vi "VCOControl-HWTimedLoop.vi"() -> ()   [LabVIEW 2014]
uses:
  <vilib>/DAQmx/create/channels.llb/DAQmx Create Channel (AI-Voltage-Basic).vi
  <vilib>/DAQmx/configure/timing.llb/DAQmx Timing (Sample Clock).vi
  <vilib>/DAQmx/read.llb/DAQmx Read (Analog Wfm 1Chan NSamp).vi
  <vilib>/DAQmx/create/channels.llb/DAQmx Create Channel (AO-Voltage-Basic).vi
  <vilib>/DAQmx/write.llb/DAQmx Write (Analog DBL 1Chan 1Samp).vi
  <vilib>/measure/NI_MAPro.lvlib
  <vilib>/measure/matone.llb/Extract Single Tone Information 1 Chan.vi
  <vilib>/addons/control/pid/NI_PID_pid.lvlib
  <vilib>/addons/control/pid/pid.llb/PID (DBL).vi
  <vilib>/platform/TimedLoop/XDataNode/XDataNode.xnode
  <vilib>/Platform/TimedLoop/XDataNode/nitl_modes.ctl
  <vilib>/Platform/TimedLoop/XDataNode/XDNodeRunTimeDep.lvlib
  <vilib>/Platform/TimedLoop/XDataNode/wakeup.ctl
  <vilib>/Platform/TimedLoop/XDataNode/timing_clust.ctl
  <vilib>/UPVI/lvhdf5/file.llb/LVH5F Operation.ctl
  <vilib>/UPVI/lvhdf5/library.llb/HDF5 Ref.ctl
  <vilib>/UPVI/lvhdf5/dataset.llb/LVH5D Operation.ctl
  <vilib>/UPVI/lvhdf5/dataset.llb/Simple OpenCreateReplace Dataset.xnode
  <vilib>/UPVI/lvhdf5/dataset.llb/Simple OpenCreateReplace Dataset (Variant).vi
  <vilib>/UPVI/lvhdf5/dataset.llb/Append Element(s) to Dataset.xnode
  <vilib>/UPVI/lvhdf5/dataset.llb/Append Element(s) to Dataset (Variant).vi
panel:
  in  "Dataset Path":string
  in  "path":path
  in  "PID gains":T1={"proportional gain (Kc)"=1.0, "integral time (Ti, min)"=0.01, "derivative time (Td, min)"=0.0} {"derivative time (Td, min)" format="%.3f"; "integral time (Ti, min)" format="%.3f"; "proportional gain (Kc)" format="%.3f"}
  in  "Setpoint Frequency":dbl format="%.2f"
  in  "stop":bool
  in  "AO Channel":tag
  in  "AI Channel":tag
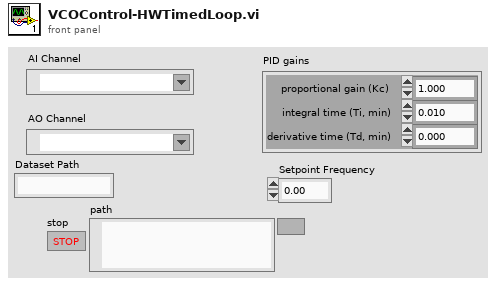
[diagram p1: front panel]
types:
  T1 = cluster{"proportional gain (Kc)":dbl, "integral time (Ti, min)":dbl, "derivative time (Td, min)":dbl}
  T2 = typedef "LVH5F Operation.ctl" = enum16{"open", "open or create", "create or replace", "create or replace (with confirmation)", "create", "open (read only)"}
  T3 = typedef "HDF5 Ref.ctl" = refnum<k1>
  T4 = typedef "XDNodeRunTimeDep.lvlib/timing_clust.ctl" = cluster{"Expected End [f-1]":u64, "Actual End [f-1]":u64, "Finished Late? [f-1]":bool, "Expected End [i-1]":u64, "Actual End [i-1]":u64, "Finished Late? [i-1]":bool, "Expected Start [i]":u64, "Actual Start [i]":u64, "Expected Start [f]":u64, "Actual Start [f]":u64, "Source Name":string, "Structure Name":string, "Period":i64, "Deadline":i64, "Offset":i64, "Start":i64, "Priority":i32, "Timeout":i32, "Mode":T5, "Wakeup Reason":T6, "Error":errorcluster, "Source Type":string, "Secondary Source Type":string, "Global End Time":u64, "Global Start Time":u64, "Frame Duration":u64, "Iteration Duration":u64, "Assigned CPU":i32, "I/O Scan Engine Mode":u32}
  T5 = typedef "XDNodeRunTimeDep.lvlib/nitl_modes.ctl" = enum32{"No Change", "Process missed periods, maintain original phase", "Discard missed periods, maintain original phase", "Process missed periods, ignore original phase", "Discard missed periods, ignore original phase"}
  T6 = typedef "XDNodeRunTimeDep.lvlib/wakeup.ctl" = enum32{"Normal", "Aborted", "Asynchronous wakeup", "Timing source error", "Timed loop error", "Timeout"}
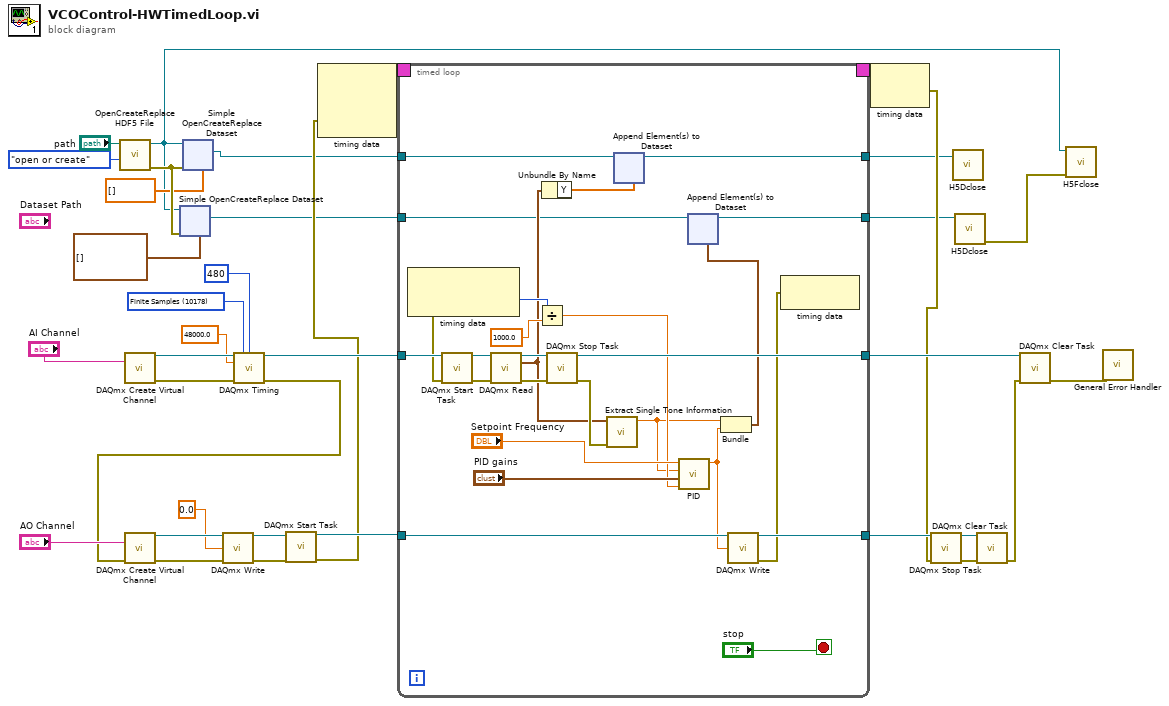
[diagram p0: block diagram]
diagram:
  w33 = 10178 items=["Finite Samples"=10178, "Continuous Samples"=10123, "Hardware Timed Single Point"=12522] ("sample mode")
  n1 = call <vilib>:"OpenCreateReplace HDF5 File.vi"("function (open or create)"=LVH5F_Operation."open or create", "path"="path") -> ("error out"=w9:errorcluster, "HDF5 Ref out"=w2:T3)  [unwired: 6 in]
  n2 = call-poly <vilib>:"DAQmx Create Virtual Channel.vi"("physical channels"="AI Channel") -> ("task out"=w35:refnum<k21>, "error out"=w34:errorcluster)  [unwired: 13 in]
  n3 = xnode "Simple OpenCreateReplace Dataset"("HDF5 Ref"=w2, "error in (no error)"=w9, "Datatype and Dataspace"=cluster{"f":dbl, "V":dbl}[] []) -> ("HDF5 Dataset Ref out"=w5:T3)  [unwired: 5 in, 2 out]
  n4 = xnode "Simple OpenCreateReplace Dataset"("HDF5 Ref"=w2, "error in (no error)"=w9, "Datatype and Dataspace"=dbl[] []) -> ("HDF5 Dataset Ref out"=w6:T3)  [unwired: 5 in, 2 out]
  n5 = call-poly <vilib>:"DAQmx Timing.vi"("task/channels in"=w35, "sample mode"=w33, "samples per channel"=480, "rate"=48000.0, "error in"=w34) -> ("task out"=w30:refnum<k21>, "error out"=w17:errorcluster)  [unwired: 9 in]
  n6 = call-poly <vilib>:"DAQmx Create Virtual Channel.vi"("physical channels"="AO Channel", "error in"=w17) -> ("task out"=w22:refnum<k21>, "error out"=w20:errorcluster)  [unwired: 12 in]
  n7 = call-poly <vilib>:"DAQmx Write.vi"("task/channels in"=w22, "data"=0.0, "error in"=w20) -> ("task out"=w21:refnum<k21>, "error out"=w19:errorcluster)  [unwired: 10 in, 1 out]
  n8 = call <vilib>:"DAQmx Start Task.vi"("task/channels in"=w21, "error in"=w19) -> ("task out"=w26:refnum<k21>, "error out"=w13:errorcluster)  [unwired: 12 in]
  n9 = node-c288(w13) -> (w15:T4)  [unwired: 2 in]
  n10 = timed-loop {
    tunnel: w30 -> [w62]
    tunnel: [w57] -> w29
    tunnel: w26 -> [w56]
    tunnel: [w55] -> w25
    timing: w15 -> [_]
    timing-out: [_] -> w14
    tunnel: w6 -> [w45]
    tunnel: w5 -> [w42]
    tunnel: [w38] -> w4
    tunnel: [w37] -> w3
    stop <- "stop" stop-if-true
    n11 = node-c288() -> (w51:errorcluster, w48:i64)  [unwired: 1 in]
    n12 = call <vilib>:"DAQmx Start Task.vi"("task/channels in"=w62, "error in"=w51) -> ("task out"=w61:refnum<k21>, "error out"=w60:errorcluster)  [unwired: 12 in]
    n13 = call-poly <vilib>:"DAQmx Read.vi"("task/channels in"=w61, "error in"=w60) -> ("task out"=w59:refnum<k21>, "data"=w44:waveform(dbl), "error out"=w58:errorcluster)  [unwired: 11 in]
    n14 = Divide(x=w48, y=1000.0 ("dt (s)")) -> (x/y=w46:dbl)
    n15 = Unbundle By Name(w44) -> ("Y"=w43:dbl[])
    n16 = call <vilib>:"DAQmx Stop Task.vi"("task/channels in"=w59, "error in"=w58) -> ("task out"=w57:refnum<k21>, "error out"=w54:errorcluster)  [unwired: 12 in]
    n17 = call-poly <vilib>:"Extract Single Tone Information.vi"("error in (no error)"=w54, "time signal in"=w44) -> ("detected frequency"=w41:dbl)  [unwired: 4 in, 5 out]
    n18 = xnode "Append Element(s) to Dataset"("HDF5 Dataset Ref"=w45, "Data Element(s)"=w43) -> ("HDF5 Dataset out"=w38:T3)  [unwired: 2 in, 3 out]
    n19 = call-poly <vilib>:"PID.vi"("dt (s)"=w46, "PID gains"="PID gains", "process variable"=w41, "setpoint"="Setpoint Frequency") -> ("output"=w40:dbl)  [unwired: 6 in, 1 out]
    n20 = Bundle("detected frequency"=w41, "output"=w40) -> (w39:cluster{"detected frequency":dbl, "output":dbl})  [unwired: 1 in]
    n21 = xnode "Append Element(s) to Dataset"("HDF5 Dataset Ref"=w42, "Data Element(s)"=w39) -> ("HDF5 Dataset out"=w37:T3)  [unwired: 2 in, 3 out]
    n22 = call-poly <vilib>:"DAQmx Write.vi"("task/channels in"=w56, "data"=w40) -> ("task out"=w55:refnum<k21>, "error out"=w50:errorcluster)  [unwired: 11 in, 1 out]
    n23 = node-c288(w50) -> ()  [unwired: 1 out]
  }
  n24 = node-c288(w14) -> (w12:errorcluster)
  n25 = call <vilib>:"DAQmx Stop Task.vi"("task/channels in"=w25, "error in"=w12) -> ("task out"=w24:refnum<k21>, "error out"=w23:errorcluster)  [unwired: 12 in]
  n26 = call <vilib>:"H5Dclose.vi"("HDF5 Dataset Ref"=w4) -> ()  [unwired: 8 in, 1 out]
  n27 = call <vilib>:"H5Dclose.vi"("HDF5 Dataset Ref"=w3) -> ("error out"=w1:errorcluster)  [unwired: 8 in]
  n28 = call <vilib>:"DAQmx Clear Task.vi"("task in"=w24, "error in"=w23) -> ("error out"=w16:errorcluster)  [unwired: 13 in]
  n29 = call <vilib>:"DAQmx Clear Task.vi"("task in"=w29, "error in"=w16) -> ("error out"=w28:errorcluster)  [unwired: 13 in]
  n30 = call <vilib>:"H5Fclose.vi"("error in (no error)"=w1, "HDF5 Ref"=w2) -> ()  [unwired: 7 in, 1 out]
  n31 = call <vilib>:"General Error Handler.vi"("error in (no error)"=w28) -> ()  [unwired: 10 in, 5 out]
